vi "Replace VI Item.vi"(5 "Class Name":string, 7 "Traverse Target":T1, 8 "error in (no error)":errorcluster, 10 "Replacement Config String":string, 11 "Assert VI Path":path) -> (0 "error out":errorcluster)   [LabVIEW 2018, in "Test.lvclass"]
doc: "Replaces a vi item as specified by a config string"
uses:
  Test.lvclass
  <vilib>/Utility/traverseref.llb/TRef TravTarget.ctl
  <vilib>/Utility/error.llb/Error Cluster From Error Code.vi
  <vilib>/ErrorRing/Error Ring.xnode
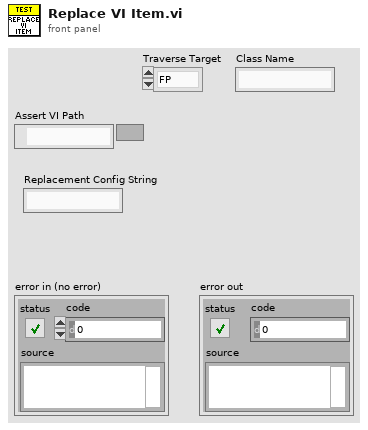
[diagram p1: front panel]
types:
  T1 = typedef "TRef TravTarget.ctl" = enum16{"FP", "BD", "Other"}
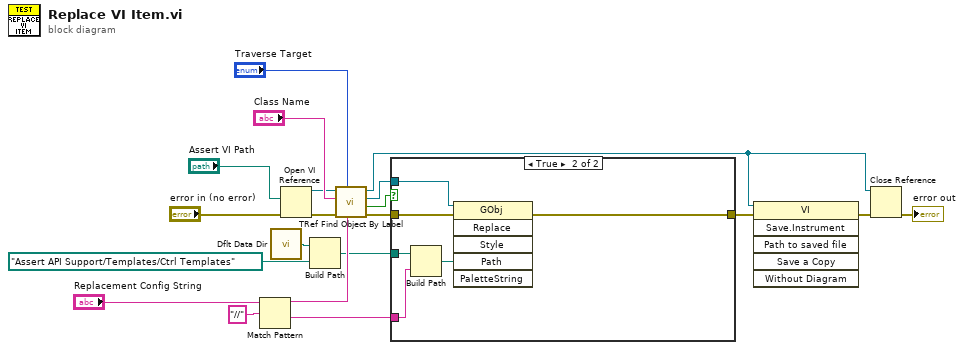
[diagram p0: block diagram]
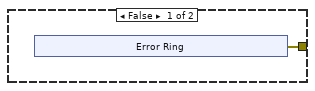
[diagram p2: hidden frame]
diagram:
  n1 = Match Pattern(string="Replacement Config String", regular expression="//") -> (before substring=w19:string, after substring=w20:string)  [unwired: 1 in, 2 out]
  n2 = call <vilib>:"Dflt Data Dir.vi"() -> ("App:Default Data Directory"=w14:path)
  n3 = Open VI Reference(vi path="Assert VI Path", error in (no error)="error in (no error)") -> (vi reference=w7:refnum<vi>, error out=w6:errorcluster)  [unwired: 4 in]
  n4 = Build Path(base path=w14, name or relative path=path "Assert API Support/Templates/Ctrl Templates" ("Path")) -> (appended path=w16:path)
  n5 = call <vilib>:"TRef Find Object By Label.vi"("Label"=w19, "Traverse Target"="Traverse Target", "error in (no error)"=w6, "Class Name"="Class Name", "VI Ref"=w7) -> ("error out"=w3:errorcluster, "Found?"=w5:bool, "Found Obj Ref"=w4:refnum<vi>, "dup VI Ref"=w2:refnum<vi>)  [unwired: 3 in]
  n6 = case shown="True" w5 {
    tunnel: w4 -> [_ w32]
    tunnel: w3 -> [_ w31]
    tunnel: [w21 w30] -> w8
    tunnel: w16 -> [_ w29]
    tunnel: w20 -> [_ w27]
    frame False {
      n7 = xnode "Error Ring"() -> ("error out"=w21:errorcluster)
    }
    frame True {
      n8 = Build Path(base path=w29, name or relative path=w27) -> (appended path=w28:path)
      n9 = invoke class="GObj" method="Replace"(reference=w32, error in=w31, "Path"=w28) -> (error out=w30:errorcluster)  [unwired: 3 in, 5 out]
    }
  }
  n10 = invoke class="VI" method="Save.Instrument"(reference=w2, error in=w8) -> (error out=w1:errorcluster)  [unwired: 4 in, 5 out]
  n11 = Close Reference(reference=w2, error in (no error)=w1) -> (error out=→"error out":errorcluster)
